vi "Receive Instrument Dataset.vi"(8 "error in (no error)":errorcluster, 10 "Instrument Dataset":cluster{"Connection":bool, "Data":dbl[]}, 11 "Test in":refnum<class "Test.lvclass">) -> (0 "error out":errorcluster, 3 "Test out":refnum<class "Test.lvclass">)   [LabVIEW 2019, in "Test.lvlib" / "Test.lvclass"]
uses:
  Test.lvclass
  Test.lvclass/Test.ctl
  Platform/Platform Messages/Get Instrument Dataset Msg/Get Instrument Data Msg.lvclass/Get Instrument Data Msg.ctl
  <vilib>/ActorFramework/Message Enqueuer/Message Enqueuer.lvclass/Message Enqueuer.ctl
  <vilib>/ActorFramework/Message Enqueuer/Enqueue.vi
  Platform/Platform Messages/Get Instrument Dataset Msg/Get Instrument Data Msg.lvclass
  C:/Program Files (x86)/National Instruments/LabVIEW 2019/vi.lib/ActorFramework/Message/Message.lvclass
  <vilib>/ActorFramework/Message Priority Queue/Priority Enqueue.vi
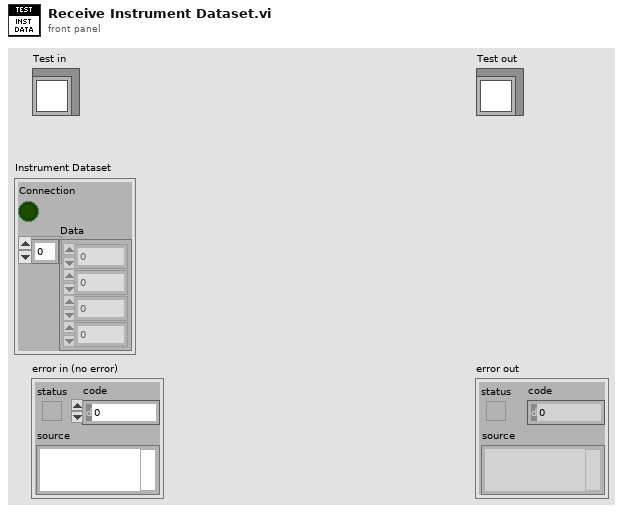
[diagram p1: front panel]
types:
  T1 = map{string, cluster{"Selected Heads":string, "Instrument":refnum<class "Message Enqueuer.lvclass">, "Platform":refnum<class "Message Enqueuer.lvclass">}}
  T2 = typedef "Test.lvlib/Cobra Data.ctl" = cluster{"M2 Dataset":cluster{"Read Temp":dbl, "Feedback":u8, "Set Temp":dbl}, "M1 Dataset":cluster{"Read Temp":dbl, "Feedback":u8, "Set Temp":dbl}, "Comp":bool}
  T3 = cluster{"Selected Heads":string, "Instrument":refnum<class "Message Enqueuer.lvclass">, "Platform":refnum<class "Message Enqueuer.lvclass">}
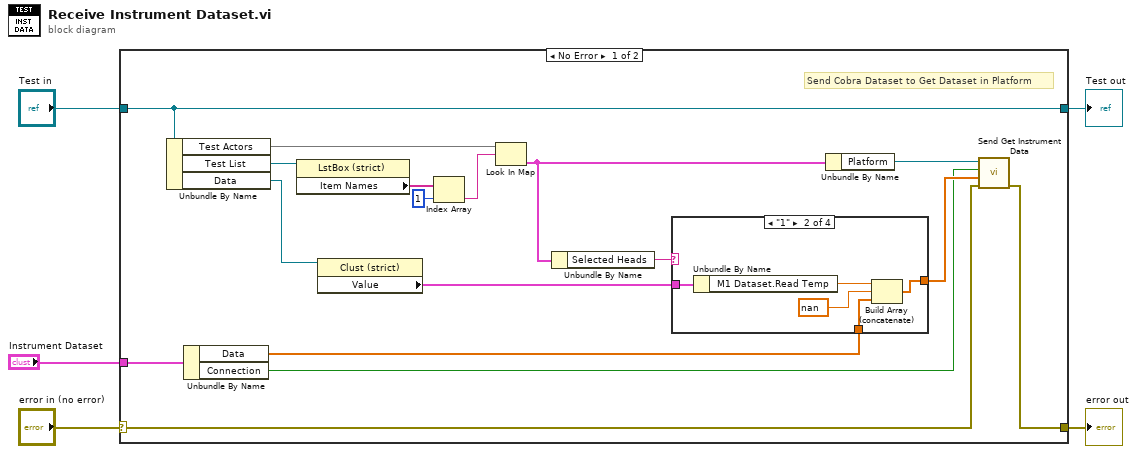
[diagram p0: block diagram]
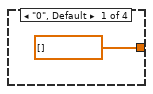
[diagram p2: hidden frame]
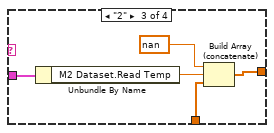
[diagram p3: hidden frame]
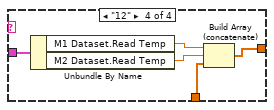
[diagram p4: hidden frame]
diagram:
  n1 = case shown="No Error" "error in (no error)" {
    selector: "error in (no error)" -> [w22 w40]
    tunnel: [w21 w40] -> w4
    tunnel: [w18 w39] -> w2
    tunnel: "Test in" -> [w18 w39]
    tunnel: "Instrument Dataset" -> [w14 _]
    frame No Error {
      # "Send Cobra Dataset to Get Dataset in Platform"
      n2 = Unbundle By Name(w18) -> ("Test Actors"=w17:T1, "Test List"=w19:refnum<vi>, "Data"=w11:refnum<vi>)
      n3 = Unbundle By Name(w14) -> ("Data"=w9:dbl[], "Connection"=w10:bool)
      n4 = property class="LstBox (strict)"(reference=w19) -> ("Item Names"=w20:string[])  [unwired: 1 in, 2 out]
      n5 = property class="Clust (strict)"(reference=w11) -> ("Value"=w13:T2)  [unwired: 1 in, 2 out]
      n6 = Index Array(array=w20, index=1) -> (element=w16:string)
      n7 = Look In Map(map=w17, key=w16) -> (value=w8:T3)  [unwired: 1 in, 1 out]
      n8 = Unbundle By Name(w8) -> ("Selected Heads"=w7:string)
      n9 = case shown="\"1\"" w7 {
        tunnel: w9 -> [_ w25 w29 w36]
        tunnel: w13 -> [_ w28 w33 w38]
        tunnel: [dbl[] [] w26 w31 w35] -> w12
        frame "0", Default {
        }
        frame "1" {
          n10 = Unbundle By Name(w28) -> ("M1 Dataset.Read Temp"=w27:dbl)
          n11 = Build Array (concatenate)(w27, nan, w25) -> (w26:dbl[])
        }
        frame "2" {
          n12 = Unbundle By Name(w33) -> ("M2 Dataset.Read Temp"=w32:dbl)
          n13 = Build Array (concatenate)(nan, w32, w29) -> (w31:dbl[])
        }
        frame "12" {
          n14 = Unbundle By Name(w38) -> ("M1 Dataset.Read Temp"=w34:dbl, "M2 Dataset.Read Temp"=w37:dbl)
          n15 = Build Array (concatenate)(w34, w37, w36) -> (w35:dbl[])
        }
      }
      n16 = Unbundle By Name(w8) -> ("Platform"=w15:refnum<class "Message Enqueuer.lvclass">)
      n17 = call "Send Get Instrument Data.vi"("error in (no error)"=w22, "Data"=w12, "Connection"=w10, "Message Enqueuer"=w15) -> ("error out"=w21:errorcluster)  [unwired: 6 in, 1 out]
    }
    frame Error {
    }
  }
  "error out" <- w4
  "Test out" <- w2
